vi "Check ECAT Installed.vi"(8 "error in (no error)":errorcluster) -> (0 "error out":errorcluster)   [LabVIEW 2020, in "SEECD System Explorer.lvlib"]
uses:
  SEECD System Explorer.lvlib
  <vilib>/registry/registry.llb/Registry SAM.ctl
  <vilib>/registry/registry.llb/Registry RtKey.ctl
  <vilib>/registry/registry.llb/Read Registry Value Simple STR.vi
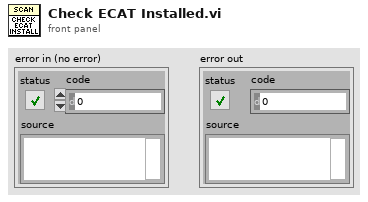
[diagram p1: front panel]
types:
  T1 = typedef "Registry SAM.ctl" = enum32{"KEY_QUERY_VALUE", "KEY_SET_VALUE", "KEY_CREATE_SUB_KEY", "KEY_ENUMERATE_SUB_KEYS", "KEY_NOTIFY", "KEY_CREATE_LINK", "KEY_READ", "KEY_WRITE", "KEY_ALL_ACCESS", "KEY_READ | KEY_WRITE"}
  T2 = typedef "Registry RtKey.ctl" = enum32{"HKEY_CLASSES_ROOT", "HKEY_CURRENT_USER", "HKEY_LOCAL_MACHINE", "HKEY_USERS", "HKEY_PERFORMANCE_DATA", "HKEY_CURRENT_CONFIG", "HKEY_DYN_DATA"}
  T3 = typedef "Registry refnum.ctl" = refnum<k1>
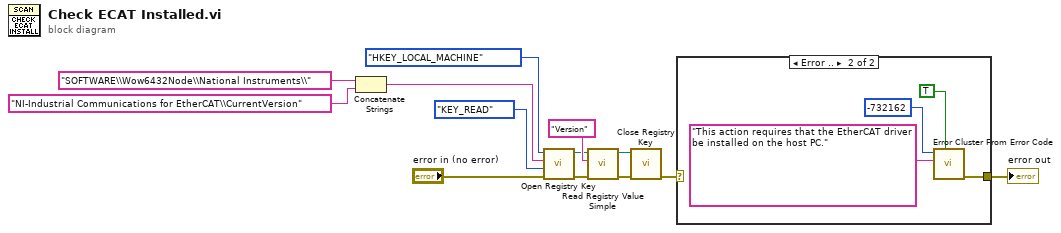
[diagram p0: block diagram]
diagram:
  n1 = Concatenate Strings("SOFTWARE\\Wow6432Node\\National Instruments\\", "NI-Industrial Communications for EtherCAT\\CurrentVersion") -> (w13:string)
  n2 = call <vilib>:"Open Registry Key.vi"("error in (no error)"="error in (no error)", "security access mask (KEY_READ | KEY_WRITE)"=Registry_SAM."KEY_READ", "subkey"=w13, "root key (HKEY_LOCAL_MACHINE)"=Registry_RtKey."HKEY_LOCAL_MACHINE") -> ("error out"=w10:errorcluster, "refnum out"=w11:T3)  [unwired: 6 in]
  n3 = call-poly <vilib>:"Read Registry Value Simple.vi"("error in (no error)"=w10, "value"="Version", "refnum"=w11) -> ("error out"=w6:errorcluster, "refnum out"=w7:T3)  [unwired: 3 in, 2 out]
  n4 = call <vilib>:"Close Registry Key.vi"("error in (no error)"=w6, "refnum"=w7) -> ("error out"=w3:errorcluster)  [unwired: 5 in]
  n5 = case shown="Error .." w3 {
    selector: w3 -> [w14 _]
    tunnel: [w14 w15] -> w4
    frame No Error {
    }
    frame Error {
      n6 = call <vilib>:"Error Cluster From Error Code.vi"("show call chain? (False)"=TRUE, "error message (\"\")"="This action requires that the EtherCAT driver be installed on the host PC." ("error message (\"\")"), "error code (0)"=-732162) -> ("error out"=w15:errorcluster)  [unwired: 6 in]
    }
  }
  "error out" <- w4
